vi "CH1_Comm_TCPIP.vi"() -> ()   [LabVIEW 2018]
uses:
  TCPIP/TCPIP.lvclass
  RxTx/RxTx.lvclass
panel:
  out "error out":errorcluster
  in  "Channel:":u16=1
  in  "RxTx.lvclass":refnum<class "RxTx.lvclass">
  in  "TCPIP.lvclass":refnum<class "TCPIP.lvclass">
  in  "remote port":u16=59041
  in  "IP":string=" 200.131.64.48"
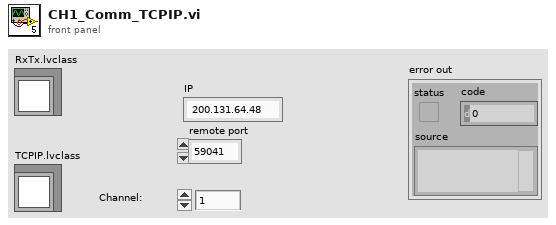
[diagram p1: front panel]
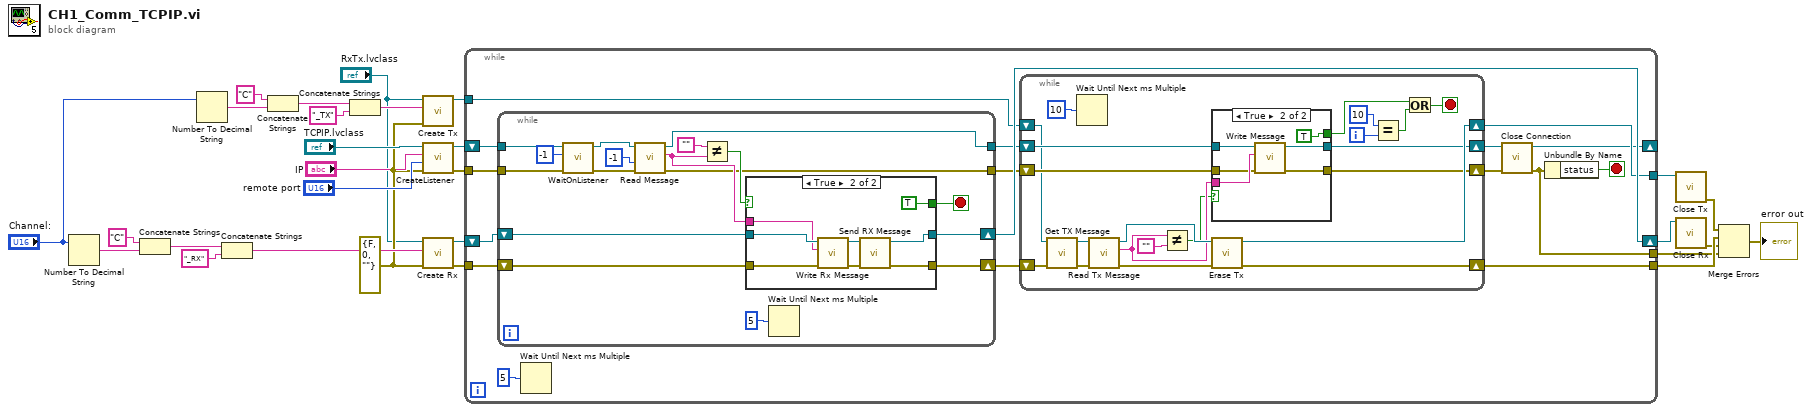
[diagram p0: block diagram]
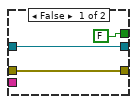
[diagram p2: hidden frame]
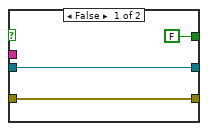
[diagram p3: hidden frame]
diagram:
  w13 = errorcluster {"status"=FALSE, "code"=0, "source"=""} ("error in")
  n1 = Number To Decimal String(number="Channel:") -> (decimal integer string=w18:string)  [unwired: 1 in]
  n2 = Concatenate Strings("C", w18) -> (w16:string)
  n3 = Number To Decimal String(number="Channel:") -> (decimal integer string=w24:string)  [unwired: 1 in]
  n4 = Concatenate Strings(w16, "_RX" ("Reader Name")) -> (w14:string)
  n5 = Concatenate Strings("C", w24) -> (w21:string)
  n6 = Concatenate Strings(w21, "_TX" ("Reader Name")) -> (w22:string)
  n7 = call "Create Tx.vi"("error in (no error)"=w13, "Writer Name"=w22, "RxTx in"="RxTx.lvclass") -> ("RxTx out"=w10:refnum<class "RxTx.lvclass">)  [unwired: 7 in, 1 out]
  n8 = call-dynamic "CreateListener.vi"("error in (no error)"=w13, "remote port"="remote port", "IP"="IP", "TCPIP in"="TCPIP.lvclass") -> ("error out"=w25:errorcluster, "TCPIP out"=w6:refnum<class "TCPIP.lvclass">)  [unwired: 6 in]
  n9 = call "Create Rx.vi"("error in (no error)"=w13, "Reader Name"=w14, "RxTx in"="RxTx.lvclass") -> ("error out"=w19:errorcluster, "RxTx out"=w9:refnum<class "RxTx.lvclass">)  [unwired: 7 in]
  n10 = while {
    tunnel: w25 -> [w45]
    tunnel: w19 -> [w44]
    tunnel: w10 -> [w30]
    shift-right: [w41] -> w8
    shift-left: w9 -> [w42]
    tunnel: [w40] -> w7
    tunnel: [w39] -> w5
    tunnel: [w32] -> w2
    shift-right: [w34] -> _
    shift-left: w6 -> [w33]
    stop <- w31 stop-if-true
    n11 = while {
      shift-right: [w80] -> w29
      shift-left: w44 -> [w92]
      shift-right: [w81] -> w41
      shift-left: w42 -> [w91]
      tunnel: w33 -> [w85]
      tunnel: w45 -> [w84]
      tunnel: [w78] -> w38
      tunnel: [w77] -> w37
      stop <- w79 stop-if-true
      n12 = call-dynamic "WaitOnListener.vi"("error in (no error)"=w84, "timeout ms"=-1, "TCPIP in"=w85) -> ("error out"=w82:errorcluster, "TCPIP out"=w83:refnum<class "TCPIP.lvclass">)  [unwired: 7 in]
      n13 = call "Read Message.vi"("error in (no error)"=w82, "timeout"=-1, "TCPIP in"=w83) -> ("error out"=w77:errorcluster, "Message"=w87:string, "TCPIP out"=w78:refnum<class "TCPIP.lvclass">)  [unwired: 6 in]
      n14 = Not Equal?(x="", y=w87) -> (x != y?=w89:bool)
      n15 = case shown="True" w89 {
        tunnel: w92 -> [w94 w101]
        tunnel: w91 -> [w95 w100]
        tunnel: [w95 w98] -> w81
        tunnel: [w94 w97] -> w80
        tunnel: w87 -> [_ w99]
        tunnel: [FALSE TRUE] -> w79
        frame False {
        }
        frame True {
          n16 = call "Write Rx Message.vi"("error in (no error)"=w101, "Rx Message"=w99, "RxTx in"=w100) -> ("error out"=w102:errorcluster, "RxTx out"=w103:refnum<class "RxTx.lvclass">)  [unwired: 7 in]
          n17 = call "Send RX Message.vi"("error in (no error)"=w102, "RxTx in"=w103) -> ("error out"=w97:errorcluster, "RxTx out"=w98:refnum<class "RxTx.lvclass">)  [unwired: 8 in]
        }
      }
      n18 = Wait Until Next ms Multiple(millisecond multiple=u32 5) -> ()  [unwired: 1 out]
    }
    n19 = Wait Until Next ms Multiple(millisecond multiple=u32 5) -> ()  [unwired: 1 out]
    n20 = while {
      shift-right: [w55] -> w36
      shift-left: w38 -> [w64]
      shift-right: [w54] -> w35
      shift-left: w37 -> [w63]
      shift-right: [w66] -> w40
      shift-left: w30 -> [w53]
      shift-right: [w65] -> w39
      shift-left: w29 -> [w52]
      i -> [w50]
      stop <- w46 stop-if-true
      n21 = call "Get TX Message.vi"("error in (no error)"=w52, "RxTx in"=w53) -> ("error out"=w62:errorcluster, "RxTx out"=w58:refnum<class "RxTx.lvclass">)  [unwired: 8 in]
      n22 = Wait Until Next ms Multiple(millisecond multiple=u32 10) -> ()  [unwired: 1 out]
      n23 = call "Read Tx Message.vi"("error in (no error)"=w62, "RxTx in"=w58) -> ("error out"=w59:errorcluster, "Tx Message"=w57:string, "RxTx out"=w60:refnum<class "RxTx.lvclass">)  [unwired: 7 in]
      n24 = Not Equal?(x=w57, y="") -> (x != y?=w56:bool)
      n25 = case shown="True" w56 {
        tunnel: w57 -> [_ w75]
        tunnel: w64 -> [w69 w74]
        tunnel: w63 -> [w68 w73]
        tunnel: [w69 w72] -> w55
        tunnel: [w68 w71] -> w54
        tunnel: [FALSE TRUE] -> w48
        frame False {
        }
        frame True {
          n26 = call "Write Message.vi"("error in (no error)"=w73, "Message"=w75, "TCPIP in"=w74) -> ("error out"=w71:errorcluster, "TCPIP out"=w72:refnum<class "TCPIP.lvclass">)  [unwired: 7 in]
        }
      }
      n27 = call "Erase Tx.vi"("error in (no error)"=w59, "RxTx in"=w60) -> ("error out"=w65:errorcluster, "RxTx out"=w66:refnum<class "RxTx.lvclass">)  [unwired: 8 in]
      n28 = Equal?(x=10, y=w50) -> (x = y?=w47:bool)
      n29 = Or(x=w48, y=w47) -> (x .or. y?=w46:bool)
    }
    n30 = call "Close Connection.vi"("error in (no error)"=w35, "TCPIP in"=w36) -> ("error out"=w32:errorcluster, "TCPIP out"=w34:refnum<class "TCPIP.lvclass">)  [unwired: 8 in]
    n31 = Unbundle By Name(w32) -> ("status"=w31:bool)
  }
  n32 = call "Close Tx.vi"("RxTx in"=w7) -> ("error out"=w3:errorcluster)  [unwired: 9 in, 1 out]
  n33 = call "Close Rx.vi"("RxTx in"=w8) -> ("error out"=w1:errorcluster)  [unwired: 9 in, 1 out]
  n34 = Merge Errors(w3, w5, w1, w2) -> (→"error out":errorcluster)
